vi "superactuator.vi"(8 "error in (no error)":errorcluster, 11 "BMC in":refnum<class "BMC.lvclass">) -> (0 "error out":errorcluster, 3 "BMC out":refnum<class "BMC.lvclass">)   [LabVIEW 2012, in "BMC.lvclass"]
uses:
  BMC.lvclass
  BMC.lvclass/BMC.ctl
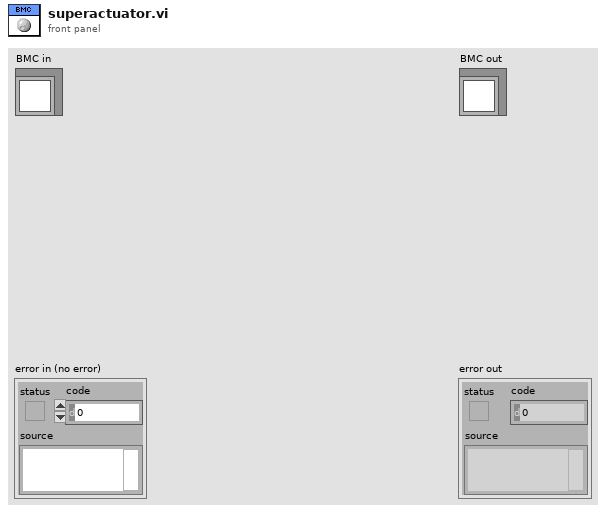
[diagram p1: front panel]
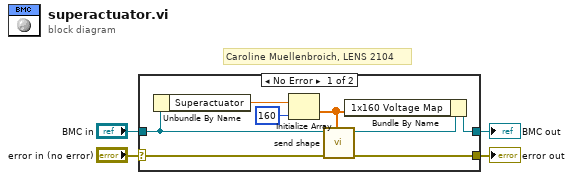
[diagram p0: block diagram]
diagram:
  # "Caroline Muellenbroich, LENS 2104"
  n1 = case shown="No Error" "error in (no error)" {
    selector: "error in (no error)" -> [w10 w14]
    tunnel: [w9 w14] -> w3
    tunnel: [w6 w13] -> w1
    tunnel: "BMC in" -> [w8 w13]
    frame No Error {
      n2 = Unbundle By Name(w8) -> ("Superactuator"=w12:dbl)
      n3 = Initialize Array(w12, 160 ("dimension size")) -> (w5:dbl[])
      n4 = call-dynamic "send shape.vi"("error in (no error)"=w10, "1x160 Voltage Map"=w5, "BMC in"=w8) -> ("error out"=w9:errorcluster, "BMC out"=w7:refnum<class "BMC.lvclass">)  [unwired: 7 in]
      n5 = Bundle By Name(cluster=w7, "1x160 Voltage Map"=w5) -> (w6:refnum<class "BMC.lvclass">)
    }
    frame Error {
    }
  }
  "error out" <- w3
  "BMC out" <- w1
